vi "Zero Pad Removal and Deinterleave.vi"(11 "Input":cdb[](array[numeric])) -> (2 "Ref":cdb[](array[numeric]), 3 "Data":cdb[](array[numeric]))   [LabVIEW 2022 SP3]
doc: "1. Removes zero padding\n2. Deinterleaves data and extracts refrence symbols"
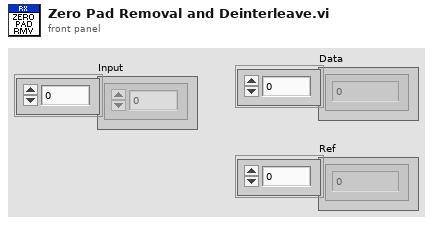
[diagram p1: front panel]
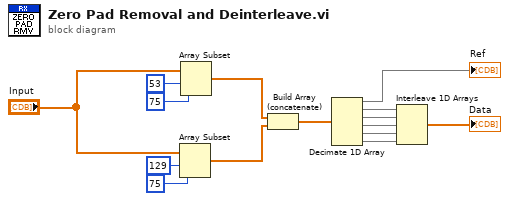
[diagram p0: block diagram]
diagram:
  n1 = Array Subset(array="Input", index=129, length=75) -> (w8:cdb[])
  n2 = Array Subset(array="Input", index=53, length=75) -> (w7:cdb[])
  n3 = Build Array (concatenate)(w7, w8) -> (w9:cdb[])
  n4 = Decimate 1D Array(w9) -> (→"Ref":cdb[], w10:cdb[], w11:cdb[], w12:cdb[], w13:cdb[], w14:cdb[])
  n5 = Interleave 1D Arrays(w10, w11, w12, w13, w14) -> (→"Data":cdb[])
